vi "Initialize Column Widths.vi"(9 "Number of Columns":i32, 11 "MCListbox Reference":refnum<vi>) -> (1 "Column Widths (Ratio)":dbl[](array[numeric]), 3 "MCListbox Reference Out":refnum<vi>)   [LabVIEW 2020, in "ListboxBusMonitor.lvlib" / "ListboxBusMonitorPanel.lvclass"]
uses:
  <vilib>/gpm_packages/@cs/BusMonitor/ListboxBusMonitor/ListboxBusMonitorPanel/ListboxBusMonitorPanel.lvclass
  <vilib>/Utility/miscctls.llb/LVRowAndColumnTypeDef.ctl
  <vilib>/gpm_packages/@cs/listbox/ListboxExtensions.lvlib
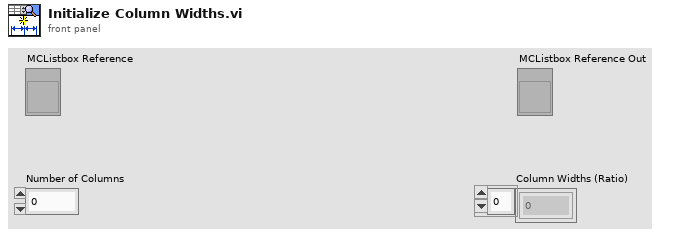
[diagram p1: front panel]
types:
  T1 = typedef "LVRowAndColumnTypeDef.ctl" = cluster{"Row":i32, "Column":i32}
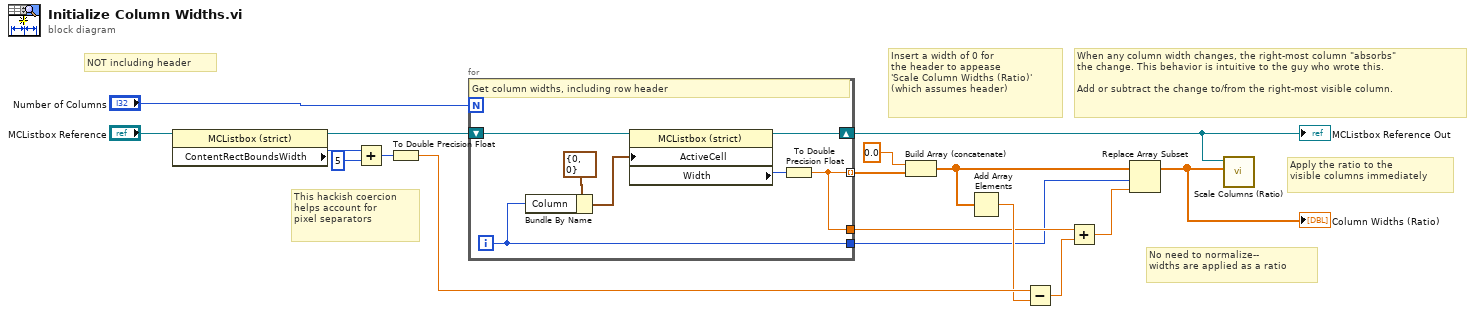
[diagram p0: block diagram]
diagram:
  # "NOT including header"
  # "Insert a width of 0 for\nthe header to appease\n'Scale Column Widths (Ratio)'\n(which assumes header)"
  # "Apply the ratio to the\nvisible columns immediately"
  # "This hackish coercion\nhelps account for\npixel separators"
  # "When any column width changes, the right-most column \"absorbs\"\nthe change. This behavior is intuitive to the guy who wrote this.\n\nAdd or subtract the change to/from the right-most visible column."
  # "No need to normalize--\nwidths are applied as a ratio"
  n1 = property class="MCListbox (strict)"(reference="MCListbox Reference") -> (reference out=w12:refnum<vi>, "ContentRectBoundsWidth"=w9:i32)  [unwired: 1 in, 1 out]
  n2 = Add(x=w9, y=5) -> (x+y=w10:i32)
  n3 = To Double Precision Float(number=w10) -> (double precision float=w17:dbl)
  n4 = for {
    N: "Number of Columns" -> [_]
    tunnel: [w20] -> w3 mode=indexing
    tunnel: [w20] -> w15
    tunnel: [w18] -> w11
    shift-right: [w19] -> w5
    shift-left: w12 -> [w24]
    i -> [w18]
    # "Get column widths, including row header"
    n5 = Bundle By Name(cluster=T1 {"Row"=0, "Column"=0} ("Active Cell:Active Cell"), "Column"=w18) -> (w22:T1)
    n6 = property class="MCListbox (strict)"(reference=w24, "ActiveCell"=w22) -> (reference out=w19:refnum<vi>, "Width"=w21:u32)  [unwired: 1 in, 1 out]
    n7 = To Double Precision Float(number=w21) -> (double precision float=w20:dbl)
  }
  "MCListbox Reference Out" <- w5
  n8 = Build Array (concatenate)(0.0, w3) -> (w2:dbl[])
  n9 = Add Array Elements(numeric array=w2) -> (sum=w16:dbl)
  n10 = Subtract(x=w17, y=w16) -> (x-y=w14:dbl)
  n11 = Add(x=w15, y=w14) -> (x+y=w13:dbl)
  n12 = Replace Array Subset(array=w2, new element=w13, index=w11) -> (w4:dbl[])
  "Column Widths (Ratio)" <- w4
  n13 = call <vilib>:"Scale Columns (Ratio).vi"("Column Widths [unitless ratio]"=w4, "MulticolumnListbox in"=w5) -> ()  [unwired: 9 in, 1 out]
